vi "Update Position.vi"(9 "Side":enum16{"Left", "Right"}(ring), 10 "Position":dbl, 11 "drive in":refnum<class "drive.lvclass">) -> (1 "Side":enum16{"Left", "Right"}(ring), 3 "drive out":refnum<class "drive.lvclass">)   [LabVIEW 2015, in "drive.lvclass"]
uses:
  drive.lvclass
  drive.lvclass/drive.ctl
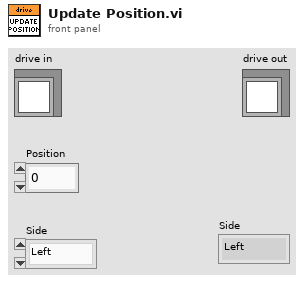
[diagram p1: front panel]
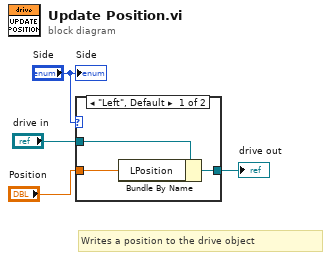
[diagram p0: block diagram]
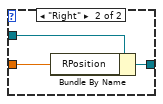
[diagram p2: hidden frame]
diagram:
  # "Writes a position to the drive object"
  n1 = case shown="\"Left\", Default" "Side" {
    tunnel: "drive in" -> [w6 w10]
    tunnel: [w5 w9] -> w3
    tunnel: "Position" -> [w7 w8]
    frame "Left", Default {
      n2 = Bundle By Name(cluster=w6, "LPosition"=w7) -> (w5:refnum<class "drive.lvclass">)
    }
    frame "Right" {
      n3 = Bundle By Name(cluster=w10, "RPosition"=w8) -> (w9:refnum<class "drive.lvclass">)
    }
  }
  "drive out" <- w3
  "Side" <- "Side"
